vi "PathPlanner_PathFinder_OpenClear.vi"() -> (3 "Open":map{i32, T1}(c390))   [LabVIEW 2019, in "PathPlanner24.lvlib"]
uses:
  PathPlanner_GridPosition_Get.vi
  PathPlanner_GridPosition_New.vi
  PathPlanner_PathFinder_Globals.vi
  PathPlanner24.lvlib
  TypeDef/PathPlannerFinderDoublePair.ctl
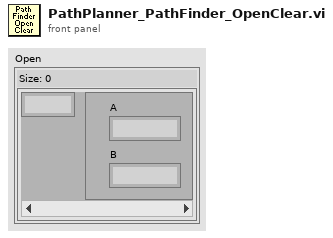
[diagram p1: front panel]
types:
  T1 = typedef "PathPlanner24.lvlib/PathPlannerFinderDoublePair.ctl" = cluster{"A":dbl, "B":dbl}
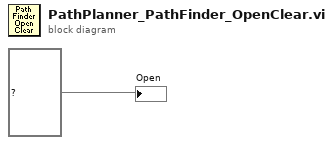
[diagram p0: block diagram]
diagram:
  "Open" <- map{i32, T1} {} ("Open")
